vi "Query.vi"(8 "error in (no error)":errorcluster, 9 "Parameters":map{string, variant}(c390), 10 "Query":string, 11 "Database Manager in":refnum<class "Database Manager.lvclass">) -> (0 "error out":errorcluster, 1 "Rows":map{string, variant}[](array[numeric]), 3 "Database Manager out":refnum<class "Database Manager.lvclass">)   [LabVIEW 2019, in "HierDAL Library.lvlib" / "Database.lvlib" / "Database Manager.lvclass"]
doc: "Executes a SQL query and retrieves the results.\nParameters are used to safely inject values into the SQL command, preventing SQL injection attacks.\nIt ensure that inputs are only ever treated as literal values and never executed.\n\nParameters can be prefixed with either :, @, or $.\ne.g.\n\"\"\"\n SELECT country, year \n FROM generals\n WHERE name = @name\n\"\"\"\n\n<b>Query</b> - The SQL query to execute.\n<b>Parameters</b> - A map of parameter (must have prefix) names and their corresponding values.\n<b>Rows</b> - A list of maps, each representing a row with column-value pairs."
uses:
  Database Manager.lvclass
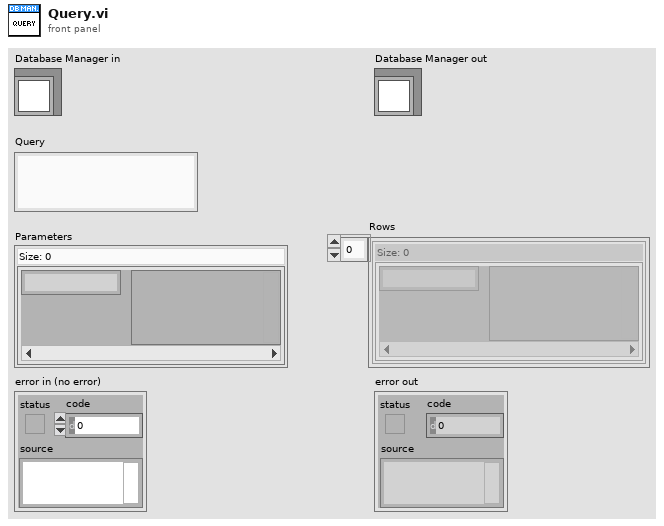
[diagram p1: front panel]
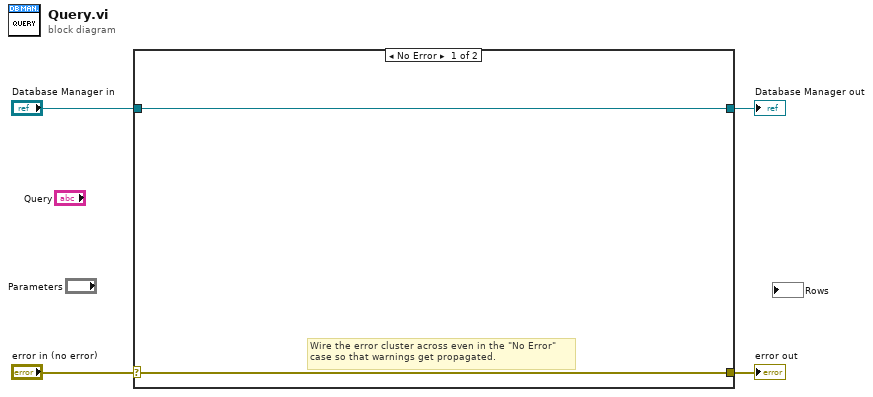
[diagram p0: block diagram]
diagram:
  n1 = case shown="No Error" "error in (no error)" {
    selector: "error in (no error)" -> [w5 w8]
    tunnel: [w5 w8] -> w3
    tunnel: [w6 w7] -> w1
    tunnel: "Database Manager in" -> [w6 w7]
    frame No Error {
      # "Wire the error cluster across even in the \"No Error\"\ncase so that warnings get propagated."
    }
    frame Error {
    }
  }
  "error out" <- w3
  "Database Manager out" <- w1
